vi "Main.vi"   [LabVIEW 2011]
types:
  T1 = typedef "WPI_DriverStationRobotMode.ctl" = enum16{"Autonomous Disabled", "Autonomous Enabled", "Teleop Disabled", "Teleop Enabled", "Timeout", "Finish"}
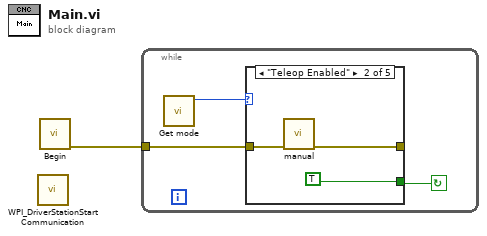
[diagram p0: block diagram]
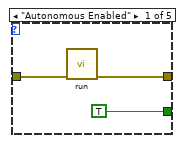
[diagram p2: hidden frame]
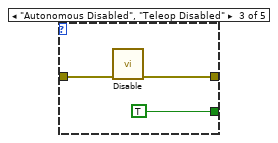
[diagram p3: hidden frame]
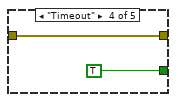
[diagram p4: hidden frame]
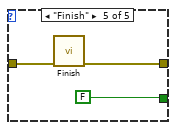
[diagram p5: hidden frame]
diagram:
  n1 = call <vilib>:"WPI_DriverStationStart Communication.vi"() -> ()  [unwired: 12 in]
  n2 = call "Begin.vi"() -> ("error out"=w1:errorcluster)  [unwired: 11 in]
  n3 = while {
    tunnel: w1 -> [w4]
    stop <- w2 continue-if-true
    n4 = call "Get mode.vi"() -> ("Robot Mode"=w3:T1)  [unwired: 11 in]
    n5 = case shown="\"Teleop Enabled\"" w3 {
      tunnel: [TRUE TRUE TRUE TRUE FALSE] -> w2
      tunnel: w4 -> [w6 w9 w12 w14 w17]
      tunnel: [w5 w8 w11 w14 w16] -> _
      frame "Autonomous Enabled" {
        n6 = call "run.vi"("error in (no error)"=w6) -> ("error out"=w5:errorcluster)  [unwired: 10 in]
      }
      frame "Teleop Enabled" {
        n7 = call "manual.vi"("error in (no error)"=w9) -> ("error out"=w8:errorcluster)  [unwired: 10 in]
      }
      frame "Autonomous Disabled", "Teleop Disabled" {
        n8 = call "Disable.vi"("error in (no error)"=w12) -> ("error out"=w11:errorcluster)  [unwired: 10 in]
      }
      frame "Timeout" {
      }
      frame "Finish" {
        n9 = call "Finish.vi"("error in (no error)"=w17) -> ("error out"=w16:errorcluster)  [unwired: 10 in]
      }
    }
  }
